vi "EndProgram.vi"(8 "error in":errorcluster, 11 "FPGA VI Reference In":refnum<k20>) -> (0 "error out":errorcluster, 3 "FPGA VI Reference Out":refnum<k20>)   [LabVIEW 2018]
uses:
  Type_Def/Type_Def Master_DataControls.ctl
  Type_Def/TypeDef_cRIODatas.ctl
  Type_Def/Type_Def IMUDatas.ctl
  Type_Def/TypeDef_BMSDatas.ctl
  Type_Def/TypeDef_BMSStatuss.ctl
  Type_Def/TypeDef FixedMotorData.ctl
  Type_Def/Type_Def Actuator Controls.ctl
  Type_Def/TypeDef_MotorData.ctl
  Type_Def/Type_Def ControlState.ctl
  Type_Def/Master_DataControl.ctl
  <vilib>/Utility/error.llb/Error Cluster From Error Code.vi
  <vilib>/rvi/errors/niLvFpgaAdjustHostInterfaceError.vi
  <vilib>/rvi/interface/nirviReadWriteControl/nirviReadWriteControl.xnode
  NiFpgaLv.dll
  <vilib>/rvi/interface/Simulation/niFpgaSimulationCallBeginRW.vi
  <vilib>/NI_Real-Time Target Support.lvlib
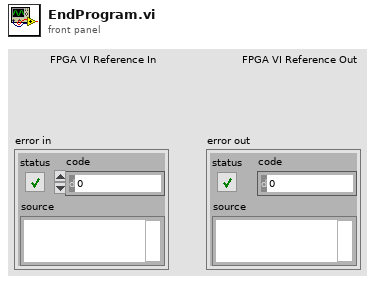
[diagram p1: front panel]
types:
  T1 = typedef "Type_Def ControlState.ctl" = enum16{"Blank", "Systems Check", "Idle", "Ready", "Pushing", "CrawlingPrecharge", "Braking", "Fault", "Boot Up", "Crawling", "Shutdown", "Service Push", "Service Wait", "Vent", "Precharge"}
  T2 = cluster{"x acceleration (g)":dbl, "Pressure (psia)":dbl, "Temperature (F)":dbl}
  T3 = typedef "Type_Def Master_DataControls.ctl" = cluster{"cRIO Data":T4, "IMU Data":T5, "BMS Data":T6, "Motor Data":T8}
  T4 = typedef "TypeDef_cRIODatas.ctl" = cluster{"HallEffect Right (cm)":dbl, "HallEffect Left (cm)":dbl, "Optical Sensor 1 (V)":dbl, "Optical Sensor 2 (V)":dbl, "24V Voltage  (V)":dbl, "24V Current (A)":dbl, "Contactor H1 Continuity":dbl, "Contactor L1 Continuity ":dbl, "Contactor H2 Continuity":dbl, "Contactor L2 Continuity ":dbl, "Brake PT(psig)":dbl, "Pump PT (psig)":dbl, "24V Temp   (C)":dbl, "Tank PT(psig) ":dbl, "ABS Pressure 1 (psig)":dbl, "ABS Pressure 2 (psig) ":dbl, "Displacement (ft)":dbl, "Velocity (ft/s)":dbl, "Time (ms)":dbl, "PV 1 Temp":dbl, "PV2 Temp":dbl}
  T5 = typedef "Type_Def IMUDatas.ctl" = cluster{"y acceleration (g)":dbl, "Pressure (psia)":dbl, "Temperature (F)":dbl}
  T6 = typedef "TypeDef_BMSDatas.ctl" = cluster{"Pack 1 Max Cell\n Voltage (V)":dbl, "Pack 1 Max Cell\n ID ":dbl, "Pack 1 Min Cell \nVoltage (V)":dbl, "Pack 1 Min Cell \nID ":dbl, "Pack 1 State of Charge  (%)":dbl, "Pack 1 Average Voltage1 (V)":dbl, "Pack 1Voltage Delta (V)":dbl, "Pack 1 Current (A)":dbl, "Pack 1 Voltage (V)":dbl, "Pack 1 Max Resistance (Ohm)":dbl, "Pack 1Min Resistance (Ohm)":dbl, "Pack 1Average Resistance (Ohm)":dbl, "Pack 1Delta Resistance (Ohm)":dbl, "Pack 1 Highest Temperature(F)":dbl, "BmsStatus1":T7, "Pack 2 Max Cell\n Voltage (V) ":dbl, "Pack 2 Max Cell\n ID  ":dbl, "Pack 2 Min Cell \nVoltage (V) ":dbl, "Pack 2 Min Cell \nID  ":dbl, "Pack 2 Average Voltage1 (V)":dbl, "Pack 2 Voltage Delta (V) ":dbl, "Pack 2 Current (A)":dbl, "Pack 2 Voltage (V) ":dbl, "Pack 2 State of Charge  (%) ":dbl, "Pack 2 Max Resistance (Ohm) ":dbl, "Pack 2 Min Resistance (Ohm)":dbl, "Pack 2 Average Resistance (Ohm)":dbl, "Pack 2 Delta Resistance (Ohm) ":dbl, "Pack 2 Highest Temperature(F) ":dbl, "BmsStatus 2":T7}
  T7 = typedef "TypeDef_BMSStatuss.ctl" = cluster{"isFault":bool, "isolationMonitoring":bool}
  T8 = typedef "TypeDef FixedMotorData.ctl" = cluster{" Velocity (RPM)":dbl, " MotorTemp(C)":dbl, " ControlTemp(C)":dbl, " DcLinkVolt(V)":dbl, " ErrorCode":dbl, "IsAlive":bool, "motorStatus":cluster{"isReady":bool, "isOn":bool, "isOperEn":bool, "isFault":bool, "isVoltEn":bool, "targetReached":bool, "isWarning":bool}, "motorControllerState":u16}
  T9 = typedef "TypeDef_MotorData.ctl" = cluster{" Velocity (RPM)":i32, " MotorTemp(C)":u8, " ControlTemp(C)":u8, " DcLinkVolt(V)":dbl, " ErrorCode":dbl, "IsAlive":bool, "motorStatus":cluster{"isReady":bool, "isOn":bool, "isOperEn":bool, "isFault":bool, "isVoltEn":bool, "targetReached":bool, "isWarning":bool}, "motorControllerState":u16}
  T10 = typedef "Type_Def Actuator Controls.ctl" = cluster{"Reverse ":bool, "Precharge Ctrl":bool, "Pump Ctrl":bool, "24 VDC Ctr":bool, "Vent Solenoid":bool, "Brake Solenoid":bool, "EMCY  Brake Solenoid":bool, "Digital Out 7B ":bool, "Forward Ctrl":bool, " Contact H2":bool, "Contact L2":bool, "LED RED":bool, "LED GREEN":bool, " Digital Out 7A":bool, " Contact H1":bool, "Contact L1":bool}
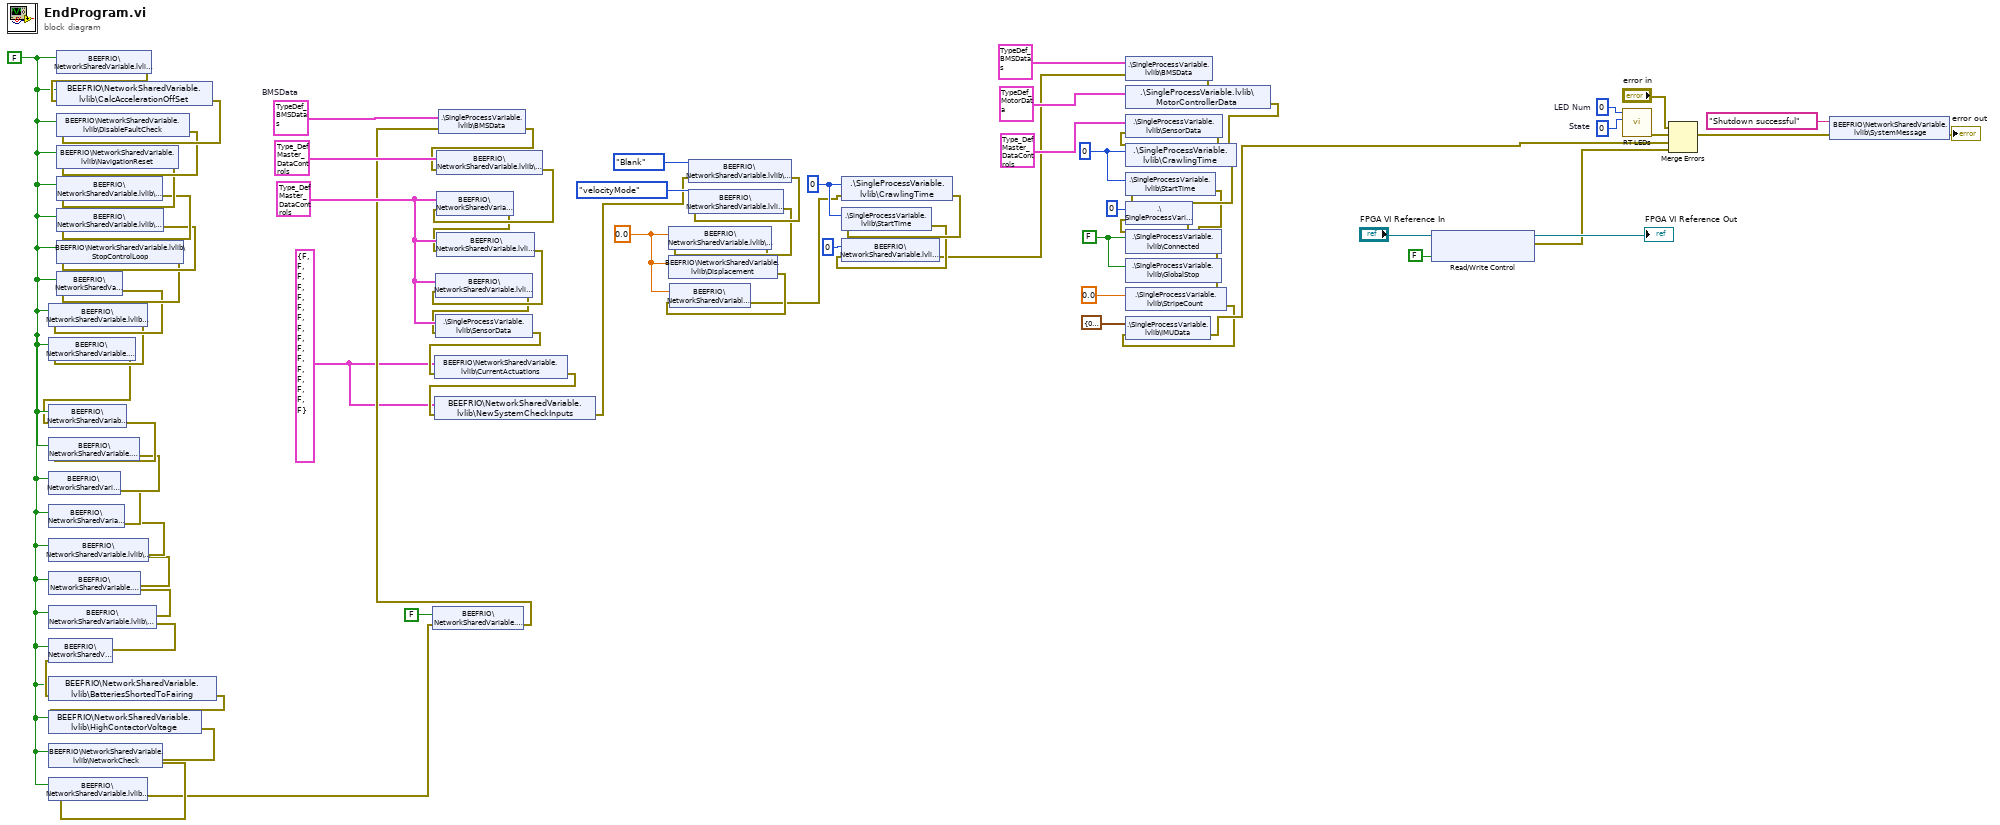
[diagram p0: block diagram]
diagram:
  w55 = 0.0 ("Acceleration")
  w59 = i64 0 ("StartTime")
  w62 = FALSE ("Connected")
  w63 = i64 0 ("CrawlingTime")
  w3 = T10 {"Reverse "=FALSE, "Precharge Ctrl"=FALSE, "Pump Ctrl"=FALSE, "24 VDC Ctr"=FALSE, "Vent Solenoid"=FALSE, "Brake Solenoid"=FALSE, "EMCY  Brake Solenoid"=FALSE, "Digital Out 7B "=FALSE, "Forward Ctrl"=FALSE, " Contact H2"=FALSE, "Contact L2"=FALSE, "LED RED"=FALSE, "LED GREEN"=FALSE, " Digital Out 7A"=FALSE, " Contact H1"=FALSE, "Contact L1"=FALSE} ("CurrentActuations")
  w66 = T3 {"cRIO Data"={"HallEffect Right (cm)"=0.0, "HallEffect Left (cm)"=0.0, "Optical Sensor 1 (V)"=0.0, "Optical Sensor 2 (V)"=0.0, "24V Voltage  (V)"=0.0, "24V Current (A)"=0.0, "Contactor H1 Continuity"=0.0, "Contactor L1 Continuity "=0.0, "Contactor H2 Continuity"=0.0, "Contactor L2 Continuity "=0.0, "Brake PT(psig)"=0.0, "Pump PT (psig)"=0.0, "24V Temp   (C)"=0.0, "Tank PT(psig) "=0.0, "ABS Pressure 1 (psig)"=0.0, "ABS Pressure 2 (psig) "=0.0, "Displacement (ft)"=0.0, "Velocity (ft/s)"=0.0, "Time (ms)"=0.0, "PV 1 Temp"=0.0, "PV2 Temp"=0.0}, "IMU Data"={"y acceleration (g)"=0.0, "Pressure (psia)"=0.0, "Temperature (F)"=0.0}, "BMS Data"={"Pack 1 Max Cell\n Voltage (V)"=0.0, "Pack 1 Max Cell\n ID "=0.0, "Pack 1 Min Cell \nVoltage (V)"=0.0, "Pack 1 Min Cell \nID "=0.0, "Pack 1 State of Charge  (%)"=0.0, "Pack 1 Average Voltage1 (V)"=0.0, "Pack 1Voltage Delta (V)"=0.0, "Pack 1 Current (A)"=0.0, "Pack 1 Voltage (V)"=0.0, "Pack 1 Max Resistance (Ohm)"=0.0, "Pack 1Min Resistance (Ohm)"=0.0, "Pack 1Average Resistance (Ohm)"=0.0, "Pack 1Delta Resistance (Ohm)"=0.0, "Pack 1 Highest Temperature(F)"=0.0, "BmsStatus1"={"isFault"=FALSE, "isolationMonitoring"=FALSE}, "Pack 2 Max Cell\n Voltage (V) "=0.0, "Pack 2 Max Cell\n ID  "=0.0, "Pack 2 Min Cell \nVoltage (V) "=0.0, "Pack 2 Min Cell \nID  "=0.0, "Pack 2 Average Voltage1 (V)"=0.0, "Pack 2 Voltage Delta (V) "=0.0, "Pack 2 Current (A)"=0.0, "Pack 2 Voltage (V) "=0.0, "Pack 2 State of Charge  (%) "=0.0, "Pack 2 Max Resistance (Ohm) "=0.0, "Pack 2 Min Resistance (Ohm)"=0.0, "Pack 2 Average Resistance (Ohm)"=0.0, "Pack 2 Delta Resistance (Ohm) "=0.0, "Pack 2 Highest Temperature(F) "=0.0, "BmsStatus 2"={"isFault"=FALSE, "isolationMonitoring"=FALSE}}, "Motor Data"={" Velocity (RPM)"=0.0, " MotorTemp(C)"=0.0, " ControlTemp(C)"=0.0, " DcLinkVolt(V)"=0.0, " ErrorCode"=0.0, "IsAlive"=FALSE, "motorStatus"={"isReady"=FALSE, "isOn"=FALSE, "isOperEn"=FALSE, "isFault"=FALSE, "isVoltEn"=FALSE, "targetReached"=FALSE, "isWarning"=FALSE}, "motorControllerState"=1}} ("AllData")
  w68 = T6 {"Pack 1 Max Cell\n Voltage (V)"=0.0, "Pack 1 Max Cell\n ID "=0.0, "Pack 1 Min Cell \nVoltage (V)"=0.0, "Pack 1 Min Cell \nID "=0.0, "Pack 1 State of Charge  (%)"=0.0, "Pack 1 Average Voltage1 (V)"=0.0, "Pack 1Voltage Delta (V)"=0.0, "Pack 1 Current (A)"=0.0, "Pack 1 Voltage (V)"=0.0, "Pack 1 Max Resistance (Ohm)"=0.0, "Pack 1Min Resistance (Ohm)"=0.0, "Pack 1Average Resistance (Ohm)"=0.0, "Pack 1Delta Resistance (Ohm)"=0.0, "Pack 1 Highest Temperature(F)"=0.0, "BmsStatus1"={"isFault"=FALSE, "isolationMonitoring"=FALSE}, "Pack 2 Max Cell\n Voltage (V) "=0.0, "Pack 2 Max Cell\n ID  "=0.0, "Pack 2 Min Cell \nVoltage (V) "=0.0, "Pack 2 Min Cell \nID  "=0.0, "Pack 2 Average Voltage1 (V)"=0.0, "Pack 2 Voltage Delta (V) "=0.0, "Pack 2 Current (A)"=0.0, "Pack 2 Voltage (V) "=0.0, "Pack 2 State of Charge  (%) "=0.0, "Pack 2 Max Resistance (Ohm) "=0.0, "Pack 2 Min Resistance (Ohm)"=0.0, "Pack 2 Average Resistance (Ohm)"=0.0, "Pack 2 Delta Resistance (Ohm) "=0.0, "Pack 2 Highest Temperature(F) "=0.0, "BmsStatus 2"={"isFault"=FALSE, "isolationMonitoring"=FALSE}}  # BMSData
  w7 = FALSE ("BMSFreeze")
  w75 = 0  # State
  w76 = 0  # LED Num
  n1 = shared-variable "BEEFRIO\\NetworkSharedVariable.lvlib\\BMSFreeze"(w7) -> (error out=w52:errorcluster)  [unwired: 1 in]
  n2 = shared-variable "BEEFRIO\\NetworkSharedVariable.lvlib\\CalcAccelerationOffSet"(w7, error in=w52) -> (error out=w51:errorcluster)
  n3 = shared-variable "BEEFRIO\\NetworkSharedVariable.lvlib\\DisableFaultCheck"(w7, error in=w51) -> (error out=w50:errorcluster)
  n4 = shared-variable "BEEFRIO\\NetworkSharedVariable.lvlib\\NavigationReset"(w7, error in=w50) -> (error out=w49:errorcluster)
  n5 = shared-variable "BEEFRIO\\NetworkSharedVariable.lvlib\\ReIntStreams"(w7, error in=w49) -> (error out=w48:errorcluster)
  n6 = shared-variable "BEEFRIO\\NetworkSharedVariable.lvlib\\SimulateData"(w7, error in=w48) -> (error out=w47:errorcluster)
  n7 = shared-variable "BEEFRIO\\NetworkSharedVariable.lvlib\\StopControlLoop"(w7, error in=w47) -> (error out=w46:errorcluster)
  n8 = shared-variable "BEEFRIO\\NetworkSharedVariable.lvlib\\Fault"(w7, error in=w46) -> (error out=w45:errorcluster)
  n9 = shared-variable "BEEFRIO\\NetworkSharedVariable.lvlib\\driveEnable"(w7, error in=w45) -> (error out=w44:errorcluster)
  n10 = shared-variable "BEEFRIO\\NetworkSharedVariable.lvlib\\ForceIdle"(w7, error in=w44) -> (error out=w1:errorcluster)
  n11 = shared-variable "BEEFRIO\\NetworkSharedVariable.lvlib\\Launch"(w7, error in=w1) -> (error out=w43:errorcluster)
  n12 = shared-variable "BEEFRIO\\NetworkSharedVariable.lvlib\\Precharge"(w7, error in=w43) -> (error out=w42:errorcluster)
  n13 = shared-variable "BEEFRIO\\NetworkSharedVariable.lvlib\\Ready"(w7, error in=w42) -> (error out=w41:errorcluster)
  n14 = shared-variable "BEEFRIO\\NetworkSharedVariable.lvlib\\Service"(w7, error in=w41) -> (error out=w40:errorcluster)
  n15 = shared-variable "BEEFRIO\\NetworkSharedVariable.lvlib\\ServicePush"(w7, error in=w40) -> (error out=w39:errorcluster)
  n16 = shared-variable "BEEFRIO\\NetworkSharedVariable.lvlib\\Shutdown"(w7, error in=w39) -> (error out=w38:errorcluster)
  n17 = shared-variable "BEEFRIO\\NetworkSharedVariable.lvlib\\SystemCheck"(w7, error in=w38) -> (error out=w37:errorcluster)
  n18 = shared-variable "BEEFRIO\\NetworkSharedVariable.lvlib\\Vent"(w7, error in=w37) -> (error out=w11:errorcluster)
  n19 = shared-variable "BEEFRIO\\NetworkSharedVariable.lvlib\\BatteriesShortedToFairing"(w7, error in=w11) -> (error out=w10:errorcluster)
  n20 = shared-variable "BEEFRIO\\NetworkSharedVariable.lvlib\\HighContactorVoltage"(w7, error in=w10) -> (error out=w9:errorcluster)
  n21 = shared-variable "BEEFRIO\\NetworkSharedVariable.lvlib\\NetworkCheck"(w7, error in=w9) -> (error out=w8:errorcluster)
  n22 = shared-variable "BEEFRIO\\NetworkSharedVariable.lvlib\\driveEnable"(w7, error in=w8) -> (error out=w5:errorcluster)
  n23 = shared-variable "BEEFRIO\\NetworkSharedVariable.lvlib\\ReintCAN"(FALSE ("ReintCAN"), error in=w5) -> (error out=w4:errorcluster)
  n24 = shared-variable ".\\SingleProcessVariable.lvlib\\BMSData"(w68, error in=w4) -> (error out=w36:errorcluster)
  n25 = shared-variable "BEEFRIO\\NetworkSharedVariable.lvlib\\DataOverride"(T3 {"cRIO Data"={"HallEffect Right (cm)"=0.0, "HallEffect Left (cm)"=0.0, "Optical Sensor 1 (V)"=0.0, "Optical Sensor 2 (V)"=0.0, "24V Voltage  (V)"=0.0, "24V Current (A)"=0.0, "Contactor H1 Continuity"=0.0, "Contactor L1 Continuity "=0.0, "Contactor H2 Continuity"=0.0, "Contactor L2 Continuity "=0.0, "Brake PT(psig)"=0.0, "Pump PT (psig)"=0.0, "24V Temp   (C)"=0.0, "Tank PT(psig) "=0.0, "ABS Pressure 1 (psig)"=0.0, "ABS Pressure 2 (psig) "=0.0, "Displacement (ft)"=0.0, "Velocity (ft/s)"=0.0, "Time (ms)"=0.0, "PV 1 Temp"=0.0, "PV2 Temp"=0.0}, "IMU Data"={"y acceleration (g)"=0.0, "Pressure (psia)"=0.0, "Temperature (F)"=0.0}, "BMS Data"={"Pack 1 Max Cell\n Voltage (V)"=0.0, "Pack 1 Max Cell\n ID "=0.0, "Pack 1 Min Cell \nVoltage (V)"=0.0, "Pack 1 Min Cell \nID "=0.0, "Pack 1 State of Charge  (%)"=0.0, "Pack 1 Average Voltage1 (V)"=0.0, "Pack 1Voltage Delta (V)"=0.0, "Pack 1 Current (A)"=0.0, "Pack 1 Voltage (V)"=0.0, "Pack 1 Max Resistance (Ohm)"=0.0, "Pack 1Min Resistance (Ohm)"=0.0, "Pack 1Average Resistance (Ohm)"=0.0, "Pack 1Delta Resistance (Ohm)"=0.0, "Pack 1 Highest Temperature(F)"=0.0, "BmsStatus1"={"isFault"=FALSE, "isolationMonitoring"=FALSE}, "Pack 2 Max Cell\n Voltage (V) "=0.0, "Pack 2 Max Cell\n ID  "=0.0, "Pack 2 Min Cell \nVoltage (V) "=0.0, "Pack 2 Min Cell \nID  "=0.0, "Pack 2 Average Voltage1 (V)"=0.0, "Pack 2 Voltage Delta (V) "=0.0, "Pack 2 Current (A)"=0.0, "Pack 2 Voltage (V) "=0.0, "Pack 2 State of Charge  (%) "=0.0, "Pack 2 Max Resistance (Ohm) "=0.0, "Pack 2 Min Resistance (Ohm)"=0.0, "Pack 2 Average Resistance (Ohm)"=0.0, "Pack 2 Delta Resistance (Ohm) "=0.0, "Pack 2 Highest Temperature(F) "=0.0, "BmsStatus 2"={"isFault"=FALSE, "isolationMonitoring"=FALSE}}, "Motor Data"={" Velocity (RPM)"=0.0, " MotorTemp(C)"=0.0, " ControlTemp(C)"=0.0, " DcLinkVolt(V)"=0.0, " ErrorCode"=0.0, "IsAlive"=FALSE, "motorStatus"={"isReady"=FALSE, "isOn"=FALSE, "isOperEn"=FALSE, "isFault"=FALSE, "isVoltEn"=FALSE, "targetReached"=FALSE, "isWarning"=FALSE}, "motorControllerState"=1}} ("DataOverride"), error in=w36) -> (error out=w35:errorcluster)
  n26 = shared-variable "BEEFRIO\\NetworkSharedVariable.lvlib\\AllData"(w66, error in=w35) -> (error out=w34:errorcluster)
  n27 = shared-variable "BEEFRIO\\NetworkSharedVariable.lvlib\\AllDataMax"(w66, error in=w34) -> (error out=w33:errorcluster)
  n28 = shared-variable "BEEFRIO\\NetworkSharedVariable.lvlib\\AllDataMin"(w66, error in=w33) -> (error out=w32:errorcluster)
  n29 = shared-variable ".\\SingleProcessVariable.lvlib\\SensorData"(w66, error in=w32) -> (error out=w31:errorcluster)
  n30 = shared-variable "BEEFRIO\\NetworkSharedVariable.lvlib\\CurrentActuations"(w3, error in=w31) -> (error out=w30:errorcluster)
  n31 = shared-variable "BEEFRIO\\NetworkSharedVariable.lvlib\\NewSystemCheckInputs"(w3, error in=w30) -> (error out=w2:errorcluster)
  n32 = shared-variable "BEEFRIO\\NetworkSharedVariable.lvlib\\CurrentState"(Type_Def_ControlState."Blank" ("CurrentState"), error in=w2) -> (error out=w29:errorcluster)
  n33 = shared-variable "BEEFRIO\\NetworkSharedVariable.lvlib\\driveMode"(enum16{"velocityMode", "torqueMode", ""}."velocityMode" ("driveMode"), error in=w29) -> (error out=w28:errorcluster)
  n34 = shared-variable "BEEFRIO\\NetworkSharedVariable.lvlib\\Acceleration"(w55, error in=w28) -> (error out=w27:errorcluster)
  n35 = shared-variable "BEEFRIO\\NetworkSharedVariable.lvlib\\Displacement"(w55, error in=w27) -> (error out=w26:errorcluster)
  n36 = shared-variable "BEEFRIO\\NetworkSharedVariable.lvlib\\Velocity"(w55, error in=w26) -> (error out=w25:errorcluster)
  n37 = shared-variable ".\\SingleProcessVariable.lvlib\\CrawlingTime"(w59, error in=w25) -> (error out=w24:errorcluster)
  n38 = shared-variable ".\\SingleProcessVariable.lvlib\\StartTime"(w59, error in=w24) -> (error out=w23:errorcluster)
  n39 = shared-variable "BEEFRIO\\NetworkSharedVariable.lvlib\\driveTarget"(i16 0 ("driveTarget"), error in=w23) -> (error out=w22:errorcluster)
  n40 = shared-variable ".\\SingleProcessVariable.lvlib\\BMSData"(T6 {"Pack 1 Max Cell\n Voltage (V)"=0.0, "Pack 1 Max Cell\n ID "=0.0, "Pack 1 Min Cell \nVoltage (V)"=0.0, "Pack 1 Min Cell \nID "=0.0, "Pack 1 State of Charge  (%)"=0.0, "Pack 1 Average Voltage1 (V)"=0.0, "Pack 1Voltage Delta (V)"=0.0, "Pack 1 Current (A)"=0.0, "Pack 1 Voltage (V)"=0.0, "Pack 1 Max Resistance (Ohm)"=0.0, "Pack 1Min Resistance (Ohm)"=0.0, "Pack 1Average Resistance (Ohm)"=0.0, "Pack 1Delta Resistance (Ohm)"=0.0, "Pack 1 Highest Temperature(F)"=0.0, "BmsStatus1"={"isFault"=FALSE, "isolationMonitoring"=FALSE}, "Pack 2 Max Cell\n Voltage (V) "=0.0, "Pack 2 Max Cell\n ID  "=0.0, "Pack 2 Min Cell \nVoltage (V) "=0.0, "Pack 2 Min Cell \nID  "=0.0, "Pack 2 Average Voltage1 (V)"=0.0, "Pack 2 Voltage Delta (V) "=0.0, "Pack 2 Current (A)"=0.0, "Pack 2 Voltage (V) "=0.0, "Pack 2 State of Charge  (%) "=0.0, "Pack 2 Max Resistance (Ohm) "=0.0, "Pack 2 Min Resistance (Ohm)"=0.0, "Pack 2 Average Resistance (Ohm)"=0.0, "Pack 2 Delta Resistance (Ohm) "=0.0, "Pack 2 Highest Temperature(F) "=0.0, "BmsStatus 2"={"isFault"=FALSE, "isolationMonitoring"=FALSE}} ("BMSData"), error in=w22) -> (error out=w20:errorcluster)
  n41 = shared-variable ".\\SingleProcessVariable.lvlib\\MotorControllerData"(T9 {" Velocity (RPM)"=0, " MotorTemp(C)"=0, " ControlTemp(C)"=0, " DcLinkVolt(V)"=0.0, " ErrorCode"=0.0, "IsAlive"=FALSE, "motorStatus"={"isReady"=FALSE, "isOn"=FALSE, "isOperEn"=FALSE, "isFault"=FALSE, "isVoltEn"=FALSE, "targetReached"=FALSE, "isWarning"=FALSE}, "motorControllerState"=1} ("MotorControllerData"), error in=w20) -> (error out=w19:errorcluster)
  n42 = shared-variable ".\\SingleProcessVariable.lvlib\\SensorData"(T3 {"cRIO Data"={"HallEffect Right (cm)"=0.0, "HallEffect Left (cm)"=0.0, "Optical Sensor 1 (V)"=0.0, "Optical Sensor 2 (V)"=0.0, "24V Voltage  (V)"=0.0, "24V Current (A)"=0.0, "Contactor H1 Continuity"=0.0, "Contactor L1 Continuity "=0.0, "Contactor H2 Continuity"=0.0, "Contactor L2 Continuity "=0.0, "Brake PT(psig)"=0.0, "Pump PT (psig)"=0.0, "24V Temp   (C)"=0.0, "Tank PT(psig) "=0.0, "ABS Pressure 1 (psig)"=0.0, "ABS Pressure 2 (psig) "=0.0, "Displacement (ft)"=0.0, "Velocity (ft/s)"=0.0, "Time (ms)"=0.0, "PV 1 Temp"=0.0, "PV2 Temp"=0.0}, "IMU Data"={"y acceleration (g)"=0.0, "Pressure (psia)"=0.0, "Temperature (F)"=0.0}, "BMS Data"={"Pack 1 Max Cell\n Voltage (V)"=0.0, "Pack 1 Max Cell\n ID "=0.0, "Pack 1 Min Cell \nVoltage (V)"=0.0, "Pack 1 Min Cell \nID "=0.0, "Pack 1 State of Charge  (%)"=0.0, "Pack 1 Average Voltage1 (V)"=0.0, "Pack 1Voltage Delta (V)"=0.0, "Pack 1 Current (A)"=0.0, "Pack 1 Voltage (V)"=0.0, "Pack 1 Max Resistance (Ohm)"=0.0, "Pack 1Min Resistance (Ohm)"=0.0, "Pack 1Average Resistance (Ohm)"=0.0, "Pack 1Delta Resistance (Ohm)"=0.0, "Pack 1 Highest Temperature(F)"=0.0, "BmsStatus1"={"isFault"=FALSE, "isolationMonitoring"=FALSE}, "Pack 2 Max Cell\n Voltage (V) "=0.0, "Pack 2 Max Cell\n ID  "=0.0, "Pack 2 Min Cell \nVoltage (V) "=0.0, "Pack 2 Min Cell \nID  "=0.0, "Pack 2 Average Voltage1 (V)"=0.0, "Pack 2 Voltage Delta (V) "=0.0, "Pack 2 Current (A)"=0.0, "Pack 2 Voltage (V) "=0.0, "Pack 2 State of Charge  (%) "=0.0, "Pack 2 Max Resistance (Ohm) "=0.0, "Pack 2 Min Resistance (Ohm)"=0.0, "Pack 2 Average Resistance (Ohm)"=0.0, "Pack 2 Delta Resistance (Ohm) "=0.0, "Pack 2 Highest Temperature(F) "=0.0, "BmsStatus 2"={"isFault"=FALSE, "isolationMonitoring"=FALSE}}, "Motor Data"={" Velocity (RPM)"=0.0, " MotorTemp(C)"=0.0, " ControlTemp(C)"=0.0, " DcLinkVolt(V)"=0.0, " ErrorCode"=0.0, "IsAlive"=FALSE, "motorStatus"={"isReady"=FALSE, "isOn"=FALSE, "isOperEn"=FALSE, "isFault"=FALSE, "isVoltEn"=FALSE, "targetReached"=FALSE, "isWarning"=FALSE}, "motorControllerState"=1}} ("SensorData"), error in=w19) -> (error out=w18:errorcluster)
  n43 = shared-variable ".\\SingleProcessVariable.lvlib\\CrawlingTime"(w63, error in=w18) -> (error out=w17:errorcluster)
  n44 = shared-variable ".\\SingleProcessVariable.lvlib\\StartTime"(w63, error in=w17) -> (error out=w16:errorcluster)
  n45 = shared-variable ".\\SingleProcessVariable.lvlib\\Time"(i64 0 ("Time"), error in=w16) -> (error out=w15:errorcluster)
  n46 = shared-variable ".\\SingleProcessVariable.lvlib\\Connected"(w62, error in=w15) -> (error out=w14:errorcluster)
  n47 = shared-variable ".\\SingleProcessVariable.lvlib\\GlobalStop"(w62, error in=w14) -> (error out=w13:errorcluster)
  n48 = shared-variable ".\\SingleProcessVariable.lvlib\\StripeCount"(0.0 ("StripeCount"), error in=w13) -> (error out=w12:errorcluster)
  n49 = shared-variable ".\\SingleProcessVariable.lvlib\\IMUData"(T2 {"x acceleration (g)"=0.0, "Pressure (psia)"=0.0, "Temperature (F)"=0.0} ("IMUData"), error in=w12) -> (error out=w53:errorcluster)
  n50 = xnode "Read/Write Control"("FPGA VI Reference In"="FPGA VI Reference In", "Pet RT Watchdog"=FALSE) -> ("FPGA VI Reference Out"=→"FPGA VI Reference Out":refnum<k20>, "error out"=w69:errorcluster)  [unwired: 1 in]
  n51 = call <vilib>:"RT LEDs.vi"("State"=w75, "LED Num"=w76) -> ("error out"=w73:errorcluster)  [unwired: 4 in, 1 out]
  n52 = Merge Errors("error in", w73, w53, w69) -> (w71:errorcluster)
  n53 = shared-variable "BEEFRIO\\NetworkSharedVariable.lvlib\\SystemMessage"("Shutdown successful" ("SysMessage"), error in=w71) -> (error out=→"error out":errorcluster)
